vi "Adb Get Debug.vi"(8 "error in (no error)":errorcluster, 11 "AdbBridge in":refnum<class "AdbBridge.lvclass">) -> (0 "error out":errorcluster, 2 "dbg msg":string, 3 "AdbBridge out":refnum<class "AdbBridge.lvclass">)   [LabVIEW 2016, in "AdbBridge.lvclass"]
uses:
  AdbBridge.lvclass
  AdbBridge.lvclass/AdbBridge.ctl
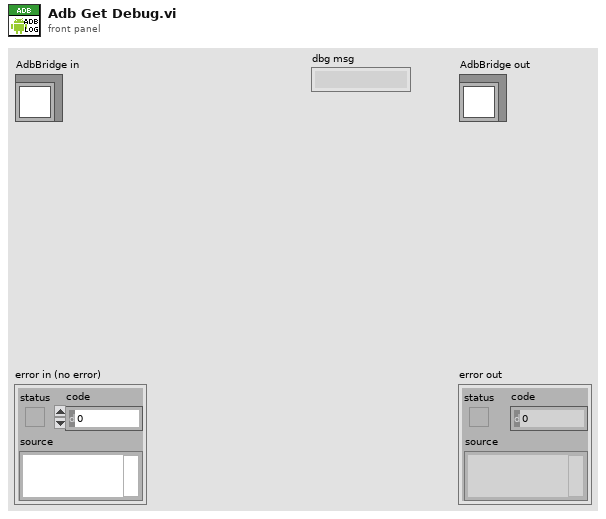
[diagram p1: front panel]
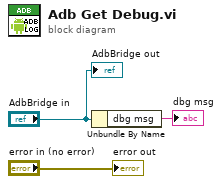
[diagram p0: block diagram]
diagram:
  n1 = Unbundle By Name("AdbBridge in") -> ("dbg msg"=→"dbg msg":string)
  "error out" <- "error in (no error)"
  "AdbBridge out" <- "AdbBridge in"
